vi "ClearBuff_re.vi"(0 "PortNumber":i32) -> (1 "String Read":string, 2 "OK Done":bool)   [LabVIEW 2016]
panel:
  # "Clear Serial Buffer"
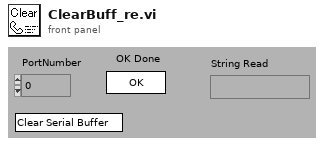
[diagram p1: front panel]
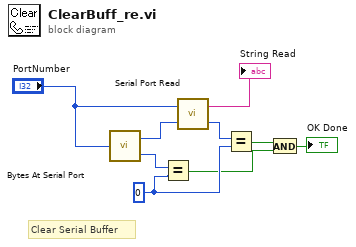
[diagram p0: block diagram]
diagram:
  w5 = 0
  # "Clear Serial Buffer"
  n1 = call <vilib>:"Bytes At Serial Port.vi"("port number"="PortNumber") -> ("byte count"=w9:u32, "error code"=w6:i32)
  n2 = Equal?(x=w6, y=w5) -> (x = y?=w3:bool)
  n3 = call <vilib>:"Serial Port Read.vi"("requested byte count"=w9, "port number"="PortNumber") -> ("error code"=w7:i32, "string read"=→"String Read":string)
  n4 = Equal?(x=w7, y=w5) -> (x = y?=w4:bool)
  n5 = And(x=w4, y=w3) -> (x .and. y?=→"OK Done":bool)
